vi "Configure Output Feedforward Parameters.vi"(6 "Feedforward Trim Limit (0)":i16 min=0 max=1000, 7 "Unit Address (1)":u8=1, 8 "error in (no error)":errorcluster, 9 "Feedforward Offset (0)":i16 min=0 max=1000, 10 "Feedforward Gain (0)":i16 min=0 max=100, 11 "VISA resource name":refnum<visa-resource-name>) -> (0 "error out":errorcluster, 3 "VISA resource name out":refnum<visa-resource-name>)   [LabVIEW 2014, in "Eurotherm 35xx Series.lvlib"]
doc: "This VI sets Feedforward parameters.\n\nNote: This VI is posible use only if Feedforward Type value (in Configure output parameters 2.vi) is \"SP\" or \"PV\"."
uses:
  <instrlib>/Eurotherm 35xx Series/Eurotherm 35xx Series.lvlib
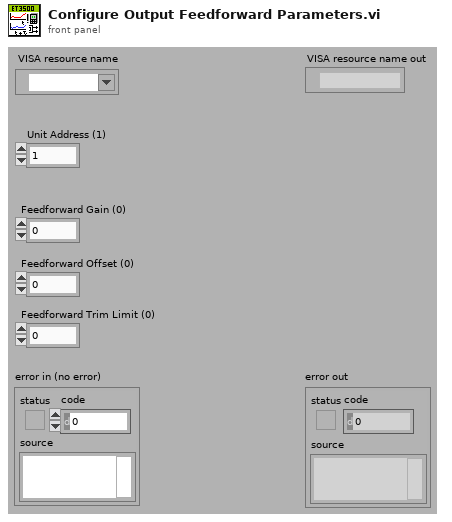
[diagram p1: front panel]
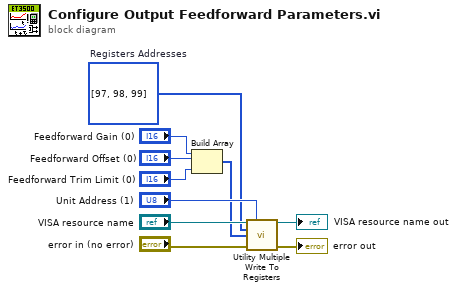
[diagram p0: block diagram]
diagram:
  w3 = u16[] [97, 98, 99]  # Registers Addresses
  n1 = Build Array("Feedforward Gain (0)", "Feedforward Offset (0)", "Feedforward Trim Limit (0)") -> (w4:i16[])
  n2 = call <instrlib>:"Utility Multiple Write To Registers.vi"("VISA resource name"="VISA resource name", "Unit Address (1)"="Unit Address (1)", "Registers Addresses (0)"=w3, "Data (0)"=w4, "error in (no error)"="error in (no error)") -> ("VISA resource name out"=→"VISA resource name out":refnum<visa-resource-name>, "error out"=→"error out":errorcluster)  [unwired: 9 in]
